vi "Unit Test expand objects on type conflict Into Sibling Error.vi"() -> ()   [LabVIEW 2019, in "Sports Unit Tests.lvclass"]
uses:
  Sports Unit Tests.lvclass
  Classes/Golf Player/Golf Player.lvclass
  C:/DSCE code/Serialization/blueserializationdemo/Test/Sports/Classes/Human/Human.lvclass
  C:/DSCE code/Serialization/blueserializationdemo/Test/Sports/Classes/Sports Player/Sports Player.lvclass
  Classes/Basketball Player/Basketball Player.lvclass
  <userlib>/Blue Origin/BlueSerialization/BlueSerializer/DeserializeOptions.ctl
  <userlib>/Blue Origin/BlueSerialization/BlueSerializer/DeserializeSlicingOptions.ctl
  <userlib>/Blue Origin/BlueSerialization/BlueSerializer/DeserializeMutationOptions.ctl
  <userlib>/Blue Origin/BlueSerialization/BlueSerializer/DeserializePreservationOptions.ctl
  <userlib>/Blue Origin/BlueSerialization/BlueSerializer/PreserveNonWiredDataOption.ctl
  Classes/Human/Human.lvclass/Human.ctl
  Classes/Sports Player/Sports Player.lvclass/Sports Player.ctl
  Classes/Golf Player/Golf Player.lvclass/Golf Player.ctl
  Classes/Human/Write Age (years).vi
  Classes/Human/Write alive_.vi
  Classes/Human/Write Height (ft).vi
  Classes/Human/Write Name.vi
  Classes/Sports Player/Write Earnings (dollars).vi
  Classes/Sports Player/Write Professional_.vi
  Classes/Sports Player/Write Sponsor.vi
  Classes/Golf Player/Write # holes in one.vi
  Classes/Golf Player/Write League.vi
  Classes/Golf Player/Write longest drive (ft).vi
  <vilib>/Utility/error.llb/Clear Errors.vi
  <vilib>/addons/_JKI Toolkits/Caraya/classes/Test/Define Test.vi
  <vilib>/addons/_JKI Toolkits/Caraya/classes/Assert/Assert Equal Value_Variant.vi
  <vilib>/addons/_JKI Toolkits/Caraya/classes/Assert/Assert Error.vi
  <vilib>/addons/_JKI Toolkits/Caraya/classes/Assert/Assert.lvclass
  <userlib>/Blue Origin/BlueSerialization/BlueSerializer/BlueSerializer.lvclass
panel:
  out "Table":string[][](table)
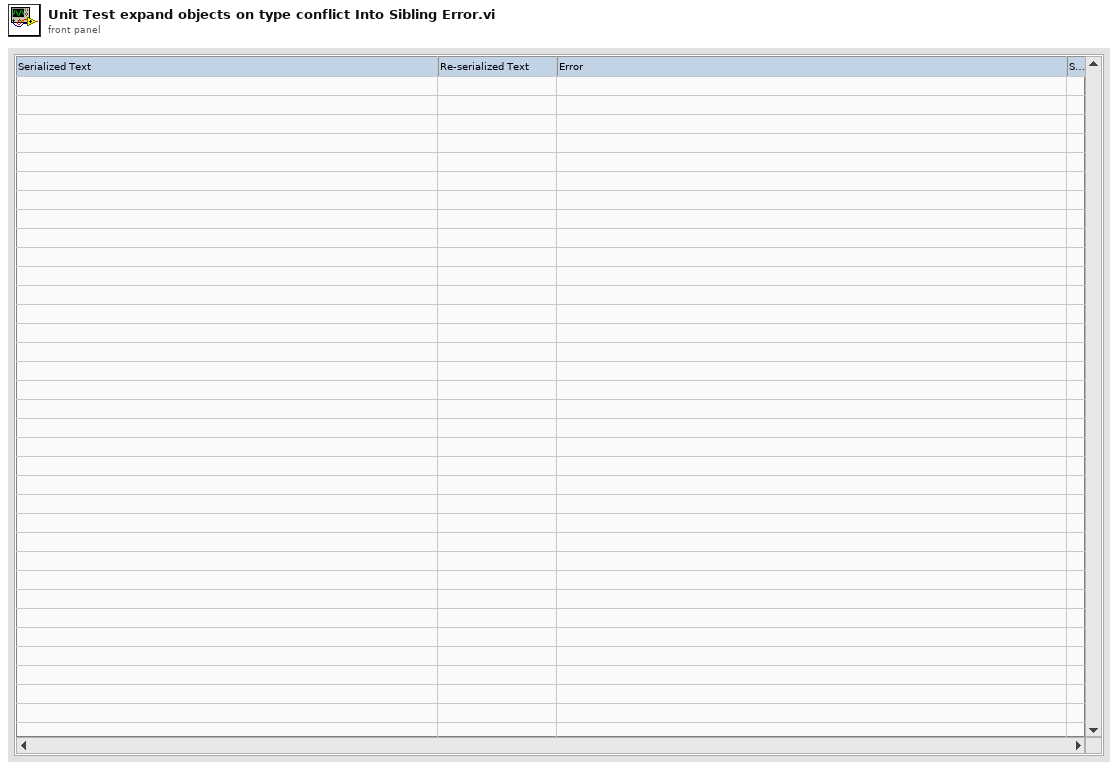
[diagram p1: front panel]
types:
  T1 = typedef "BlueSerialization.lvlib/BlueSerializer.lvclass/DeserializeOptions.ctl" = cluster{"deserialize non-BlueSerializable objects from hex?":bool, "expand objects on type conflict?":bool, "Slicing":T2, "Mutation Options":T3, "Preservation Options":T4}
  T2 = typedef "BlueSerialization.lvlib/BlueSerializer.lvclass/DeserializeSlicingOptions.ctl" = cluster{"slice flattened object data on error?":bool, "sliceable class names":string[]}
  T3 = typedef "BlueSerialization.lvlib/BlueSerializer.lvclass/DeserializeMutationOptions.ctl" = cluster{"error on inserted parent levels?":bool, "\terror on obsolete parent levels?":bool}
  T4 = typedef "BlueSerialization.lvlib/BlueSerializer.lvclass/DeserializePreservationOptions.ctl" = cluster{"Preserve wired serialized data?":bool, "Preserve wired non-serialized data":T5}
  T5 = typedef "BlueSerialization.lvlib/BlueSerializer.lvclass/PreserveNonWiredDataOption.ctl" = enum16{"Don't preserve", "Preserve (error on less-specific wired types)", "Preserve (except on less-specific wired types)"}
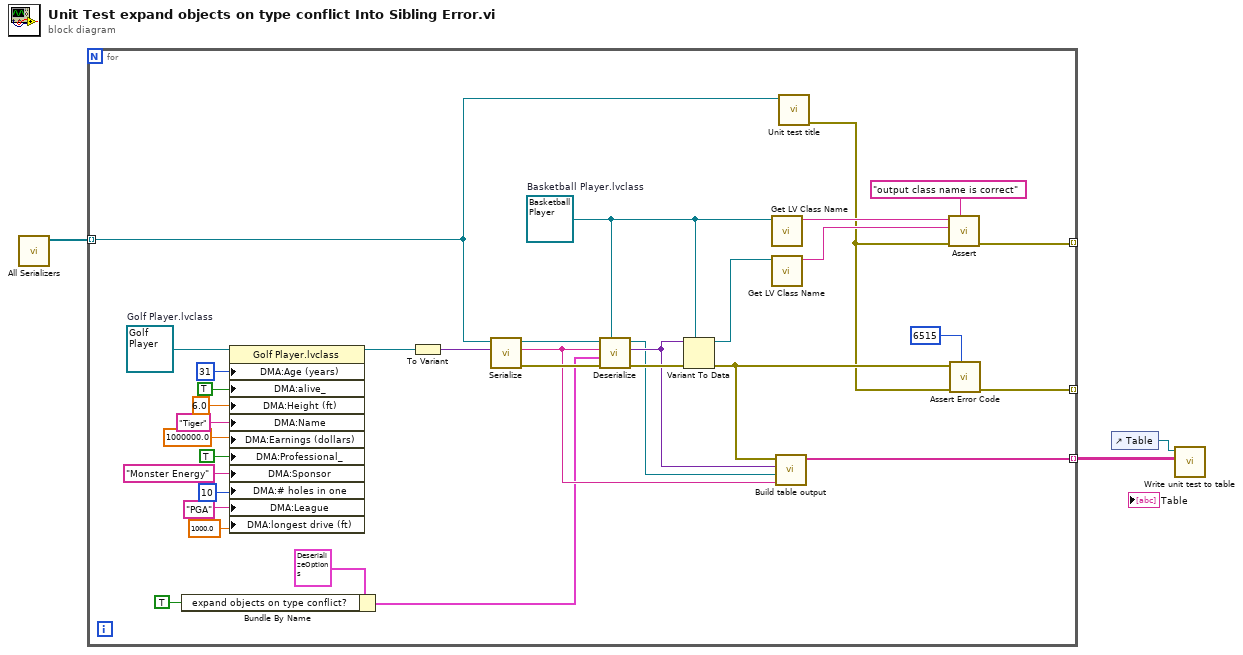
[diagram p0: block diagram]
diagram:
  n1 = call "All Serializers.vi"() -> ("All serializers"=w2:refnum<class "BlueSerializer.lvclass">[])  [unwired: 11 in]
  n2 = for {
    tunnel: w2 -> [w4] mode=indexing
    tunnel: [w9] -> _ mode=indexing
    tunnel: [w21] -> _ mode=indexing
    tunnel: [w17] -> w1 mode=indexing
    w12 = refnum<class "Basketball Player.lvclass"> refnum  # Basketball Player.lvclass
    w16 = refnum<class "Golf Player.lvclass"> refnum  # Golf Player.lvclass
    n3 = Bundle By Name(cluster=T1 {"deserialize non-BlueSerializable objects from hex?"=FALSE, "expand objects on type conflict?"=FALSE, "Slicing"={"slice flattened object data on error?"=FALSE, "sliceable class names"=[]}, "Mutation Options"={"error on inserted parent levels?"=FALSE, "\terror on obsolete parent levels?"=FALSE}, "Preservation Options"={"Preserve wired serialized data?"=FALSE, "Preserve wired non-serialized data"=enum."Don't preserve"}} ("Deserialize Options"), "expand objects on type conflict?"=TRUE ("Allow class expansion?")) -> (w5:T1)
    n4 = property on="Property Node" class="Golf Player.lvclass"(reference=w16, "DMA:Age (years)"=u16 31 ("Age (years)"), "DMA:alive_"=TRUE ("alive_"), "DMA:Height (ft)"=6.0 ("Height (ft)"), "DMA:Name"="Tiger" ("Name"), "DMA:Earnings (dollars)"=1000000.0 ("Earnings (dollars)"), "DMA:Professional_"=TRUE ("Professional_"), "DMA:Sponsor"="Monster Energy" ("Sponsor"), "DMA:# holes in one"=10 ("# holes in one"), "DMA:League"="PGA" ("Sponsor"), "DMA:longest drive (ft)"=1000.0 ("longest drive (ft)")) -> (reference out=w22:refnum<class "Golf Player.lvclass">)  [unwired: 1 in, 1 out]
    n5 = To Variant(anything=w22) -> (Variant=w35:variant)
    n6 = call <userlib>:"Serialize.vi"("Anything"=w35, "BlueSerializer in"=w4) -> ("error out"=w37:errorcluster, "Serialized Text"=w18:string, "BlueSerializer out"=w36:refnum<class "BlueSerializer.lvclass">)  [unwired: 7 in]
    n7 = call <userlib>:"Deserialize.vi"("Anything"=w12, "error in (no error)"=w37, "Deserialize Options"=w5, "Serialized Text"=w18, "BlueSerializer in"=w36) -> ("error out"=w34:errorcluster, "Variant"=w20:variant, "BlueSerializer out"=w19:refnum<class "BlueSerializer.lvclass">)  [unwired: 4 in]
    n8 = Variant To Data(error in=w34, type=w12, Variant=w20) -> (data=w33:refnum<class "Basketball Player.lvclass">, error out=w11:errorcluster)
    n9 = call <vilib>:"Get LV Class Name.vi"("object"=w12) -> ("class name"=w32:string)  [unwired: 9 in, 1 out]
    n10 = call <vilib>:"Get LV Class Name.vi"("object"=w33) -> ("class name"=w31:string)  [unwired: 9 in, 1 out]
    n11 = call "Build table output.vi"("serialized text"=w18, "BlueSerializer in"=w19, "deserialized variant"=w20, "variant to data error"=w11) -> ("table output"=w17:string[])  [unwired: 7 in]
    n12 = call "Unit test title.vi"("serializer"=w4) -> ("error out"=w10:errorcluster)  [unwired: 9 in, 1 out]
    n13 = call-poly <vilib>:"Assert.vi"("Label"="output class name is correct", "error in (no error)"=w10, "Y"=w31, "X"=w32) -> ("error out"=w21:errorcluster)  [unwired: 7 in]
    n14 = call "Assert Error Code.vi"("Assert specific error code"=6515, "error in (no error)"=w10, "Error?"=w11) -> ("error out"=w9:errorcluster)  [unwired: 8 in]
  }
  n15 = control-ref of="Table"() -> (w3:refnum<vi>)
  n16 = call "Write unit test to table.vi"("Table"=w1, "Table ref in"=w3) -> ()  [unwired: 9 in, 1 out]
